vi "Drag Over Draw.vi"(8 "error in (no error)":errorcluster, 10 "DragOver Output":T1={"Displayed Row"=0, "Position"=enum."On Row", "Row's TreeItem index"=0, "indent"=0, "Accepted?"=FALSE, "Insertion index"=0, "Top left visible TreeItem index"=0, "Bar type"=enum."tilda up"}, 11 "BetterTreeHandle in":refnum<class "BetterTreeHandle.lvclass">) -> (0 "error out":errorcluster, 3 "BetterTreeHandle out":refnum<class "BetterTreeHandle.lvclass">)   [LabVIEW 2020, in "BetterDragAndDrop.lvlib" / "BetterTreeHandle.lvclass"]
uses:
  BetterTreeHandle.lvclass
  SubVIs/DragOver Output.ctl
  SubVIs/DragOverPosition.ctl
  BetterTreeBar/SubVIs/Horizontal Bar Enumeration.ctl
  BetterTreeHandle.lvclass/BetterTreeHandle.ctl
  BetterHandle/BetterHandle.lvclass
  BetterTreeBar/BetterHorizontalBar.lvclass
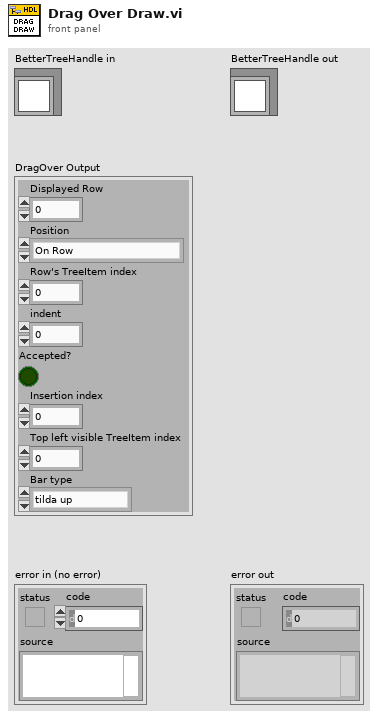
[diagram p1: front panel]
types:
  T1 = typedef "BetterDragAndDrop.lvlib/BetterHandle.lvclass/DragOver Output.ctl" = cluster{"Displayed Row":i32, "Position":T2, "Row's TreeItem index":i32, "indent":i32, "Accepted?":bool, "Insertion index":i32, "Top left visible TreeItem index":i32, "Bar type":T3}
  T2 = typedef "BetterDragAndDrop.lvlib/BetterHandle.lvclass/DragOverPosition.ctl" = enum16{"On Row", "Inbetween"}
  T3 = typedef "BetterDragAndDrop.lvlib/BetterHorizontalBar.lvclass/Horizontal Bar Enumeration.ctl" = enum16{"None", "only bar", "tilda up"}
  T4 = typedef "BetterDragAndDrop.lvlib/BetterTreeHandle.lvclass/TreeItem.ctl" = cluster{"Left Cell String":string, "Child Text":string[], "Child Tag":string, "Item Indent":i32, "Child Only?":bool, "Glyph Index":i32, "Font Color":u32}
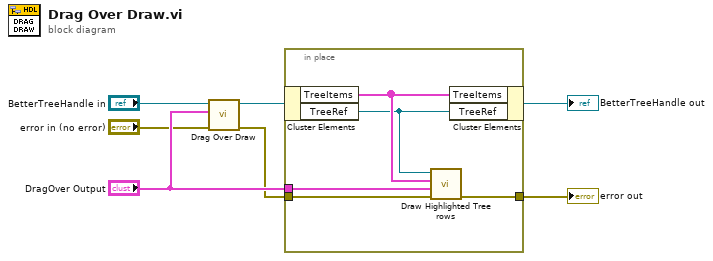
[diagram p0: block diagram]
diagram:
  n1 = call-parent "Drag Over Draw.vi"("error in (no error)"="error in (no error)", "DragOver Output"="DragOver Output", "BetterHandle in"="BetterTreeHandle in") -> ("error out"=w1:errorcluster, "BetterHandle out"=w5:refnum<class "BetterTreeHandle.lvclass">)  [unwired: 7 in]
  n2 = in-place {
    in-place-border: w1 -> [w10]
    in-place-border: [w8] -> w7
    in-place-border: "DragOver Output" -> [w9]
    n3 = in-place-cluster #1(w5) -> ("TreeItems"=w12:T4[], "TreeRef"=w11:refnum<vi>)
    n4 = call "Draw Highlighted Tree rows.vi"("error in (no error)"=w10, "DragOver Output"=w9, "TreeItems"=w12, "TreeRef"=w11) -> ("error out"=w8:errorcluster)  [unwired: 7 in]
    n5 = in-place-cluster #1("TreeItems"=w12, "TreeRef"=w11) -> (→"BetterTreeHandle out":refnum<class "BetterTreeHandle.lvclass">)
  }
  "error out" <- w7
